vi "Read Charm Splitter.vi"(8 "error in (no error)":errorcluster, 11 "MainController in":refnum<class "MainController.lvclass">) -> (0 "error out":errorcluster, 2 "Charm Splitter":refnum<vi>, 3 "MainController out":refnum<class "MainController.lvclass">)   [LabVIEW 2012, in "Win8uiFramework.lvlib" / "MainController.lvclass"]
uses:
  MainController.lvclass
  MainController.lvclass/MainController.ctl
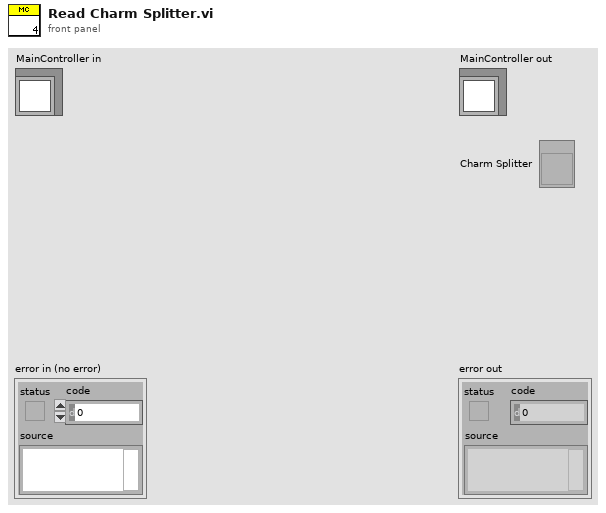
[diagram p1: front panel]
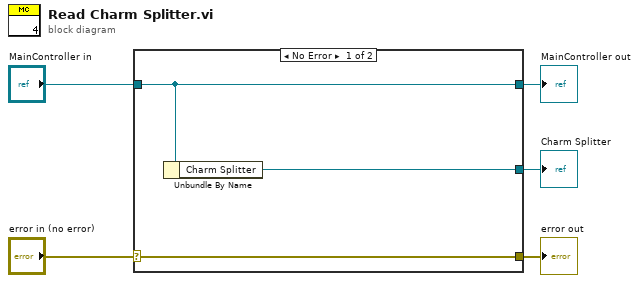
[diagram p0: block diagram]
diagram:
  n1 = case shown="No Error" "error in (no error)" {
    selector: "error in (no error)" -> [w8 w9]
    tunnel: [w8 w9] -> w4
    tunnel: [w7 w10] -> w2
    tunnel: "MainController in" -> [w7 w10]
    tunnel: [w6 _] -> w1
    frame No Error {
      n2 = Unbundle By Name(w7) -> ("Charm Splitter"=w6:refnum<vi>)
    }
    frame Error {
    }
  }
  "error out" <- w4
  "MainController out" <- w2
  "Charm Splitter" <- w1
